vi "SUB FFT.vi"(2 "Time waveform":waveform(dbl), 3 "Cluster":T2={"Windowing"=2, "log/linear\n"=enum."Linear", "display unit"=enum."Vpk"} {"Windowing" items=["Rectangle"=0, "Hanning"=1, "Hamming"=2, "Blackman-Harris"=3, "Exact Blackman"=4, "Blackman"=5, "Flat Top"=6, "4 Term B-Harris "=7, "7 Term B-Harris"=8, "Low Sidelobe"=9, "Blackman Nuttall"=11, "Triangle"=30, "Bartlett-Hanning"=31, "Bohman"=32, "Parzen"=33, "Welch"=34, "Kaiser"=60, "Dolph-Chebyshev"=61, "Gaussian"=62]}) -> (0 "Fourier Waveform":waveform(dbl))   [LabVIEW 2017]
uses:
  <vilib>/Analysis/4window.llb/windowTd.ctl
  <vilib>/Analysis/0measdsp.llb/Scaled Time Domain Window (DBL).vi
  <vilib>/Analysis/NI_AALPro.lvlib
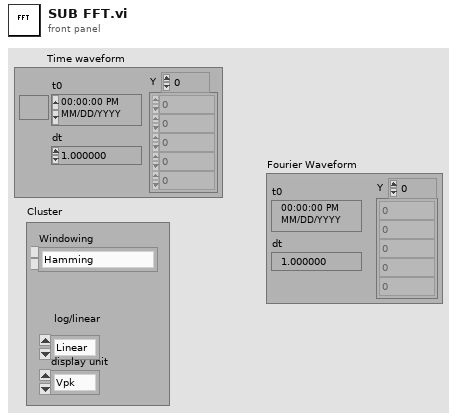
[diagram p1: front panel]
types:
  T1 = typedef "NI_AALPro.lvlib/windowTd.ctl" = u32
  T2 = cluster{"Windowing":T1, "log/linear\n":enum16{"Linear", "dB", "dBm"}, "display unit":enum32{"Vrms", "Vpk", "Vrms^2", "Vpk^2", "Vrms/rtHz", "Vpk/rtHz", "Vrms^2/Hz", "Vpk^2/Hz"}}
  T3 = enum16{"Power (Vrms^2)", "Amplitude (Vrms)", "Gain (amplitude ratio)"}
  T4 = enum32{"Vrms", "Vpk", "Vrms^2", "Vpk^2", "Vrms/rtHz", "Vpk/rtHz", "Vrms^2/Hz", "Vpk^2/Hz"}
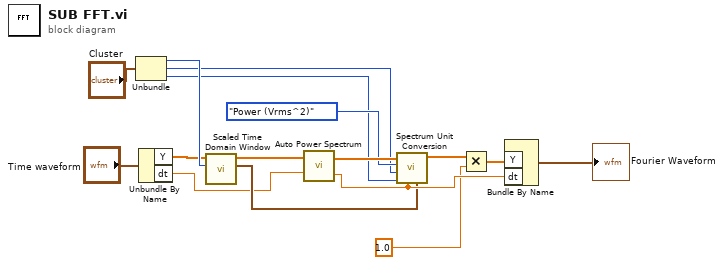
[diagram p0: block diagram]
diagram:
  n1 = Unbundle("Cluster") -> ("Windowing"=w10:T1, "log/linear"=w5:enum16{"Linear", "dB", "dBm"}, "display unit"=w4:T4)
  n2 = Unbundle By Name("Time waveform") -> ("Y"=w8:dbl[], "dt"=w7:dbl)
  n3 = call-poly <vilib>:"Scaled Time Domain Window.vi"("window"=w10, "X"=w8) -> ("window properties"=w14:cluster{"eq noise BW":dbl, "coherent gain":dbl}, "Windowed X"=w12:dbl[])  [unwired: 7 in, 1 out]
  n4 = call <vilib>:"Auto Power Spectrum.vi"("dt"=w7, "Signal (V)"=w12) -> ("df"=w15:dbl, "Power Spectrum (V^2 rms)"=w13:dbl[])
  n5 = call <vilib>:"Spectrum Unit Conversion.vi"("window constants"=w14, "df"=w15, "display unit"=w4, "log/linear"=w5, "spectrum type"=T3."Power (Vrms^2)", "Spectrum in"=w13) -> ("Spectrum out"=w2:dbl[])  [unwired: 4 in, 1 out]
  n6 = Multiply(x=w2, y=1.0) -> (x*y=w3:dbl[])
  n7 = Bundle By Name ("Build Waveform")("Y"=w3, "dt"=w15) -> (→"Fourier Waveform":waveform(dbl))  [unwired: 1 in]
